vi "Analysis.Result Summaries, First and Last Pass Yield Paretos, Metrics Table.vi"(11 "ResultSum":T2[](array[typedef])) -> (0 "To Date":timestamp, 1 "From Date":timestamp, 2 "Test Count Table":string[][](table), 3 "Failure Pareto":string[][](table), 4 "LP Times Hist":T1(graph), 5 "Metrics Table":string[][](table), 6 "FP Times Hist":T1(graph), 7 "Durs":string[][](table))   [LabVIEW 2024]
uses:
  Analysis.Result Summary.ctl
panel:
  out "Tst Cnts":i32
  out "SNs":i32
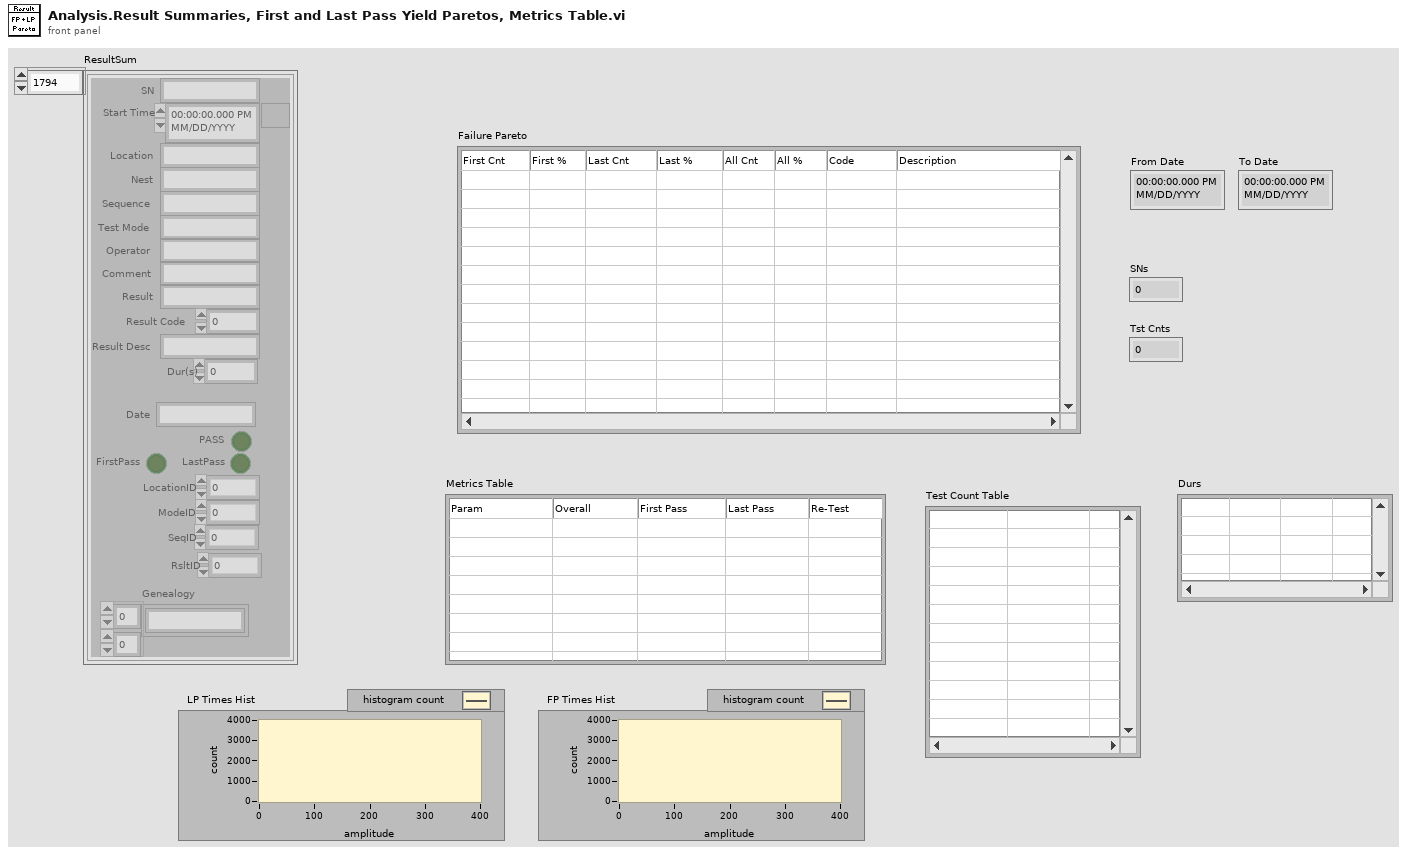
[diagram p1: front panel]
types:
  T1 = cluster{"X Values":dbl[], "Histogram: h(x)":i32[]}
  T2 = typedef "Analysis.Result Summary.ctl" = cluster{"SN":string, "Start Time":timestamp, "Location":string, "Nest":string, "Sequence":string, "Operator":string, "Test Mode":string, "Comment":string, "Result":string, "Result Code":i32, "Result Desc":string, "Date":string, "Dur(s)":dbl, "PASS":bool, "FirstPass":bool, "LastPass":bool, "LocationID":i32, "ModeID":i32, "SeqID":i32, "RsltID":i32, "Genealogy":string[][]}
  T3 = typedef "Analysis.Result Summary, Metrics.ctl" = cluster{"Pass Cnt":i32, "Fail Cnt":i32, "Yield%":dbl, "Test Cnt":i32, "SN Cnt":i32}
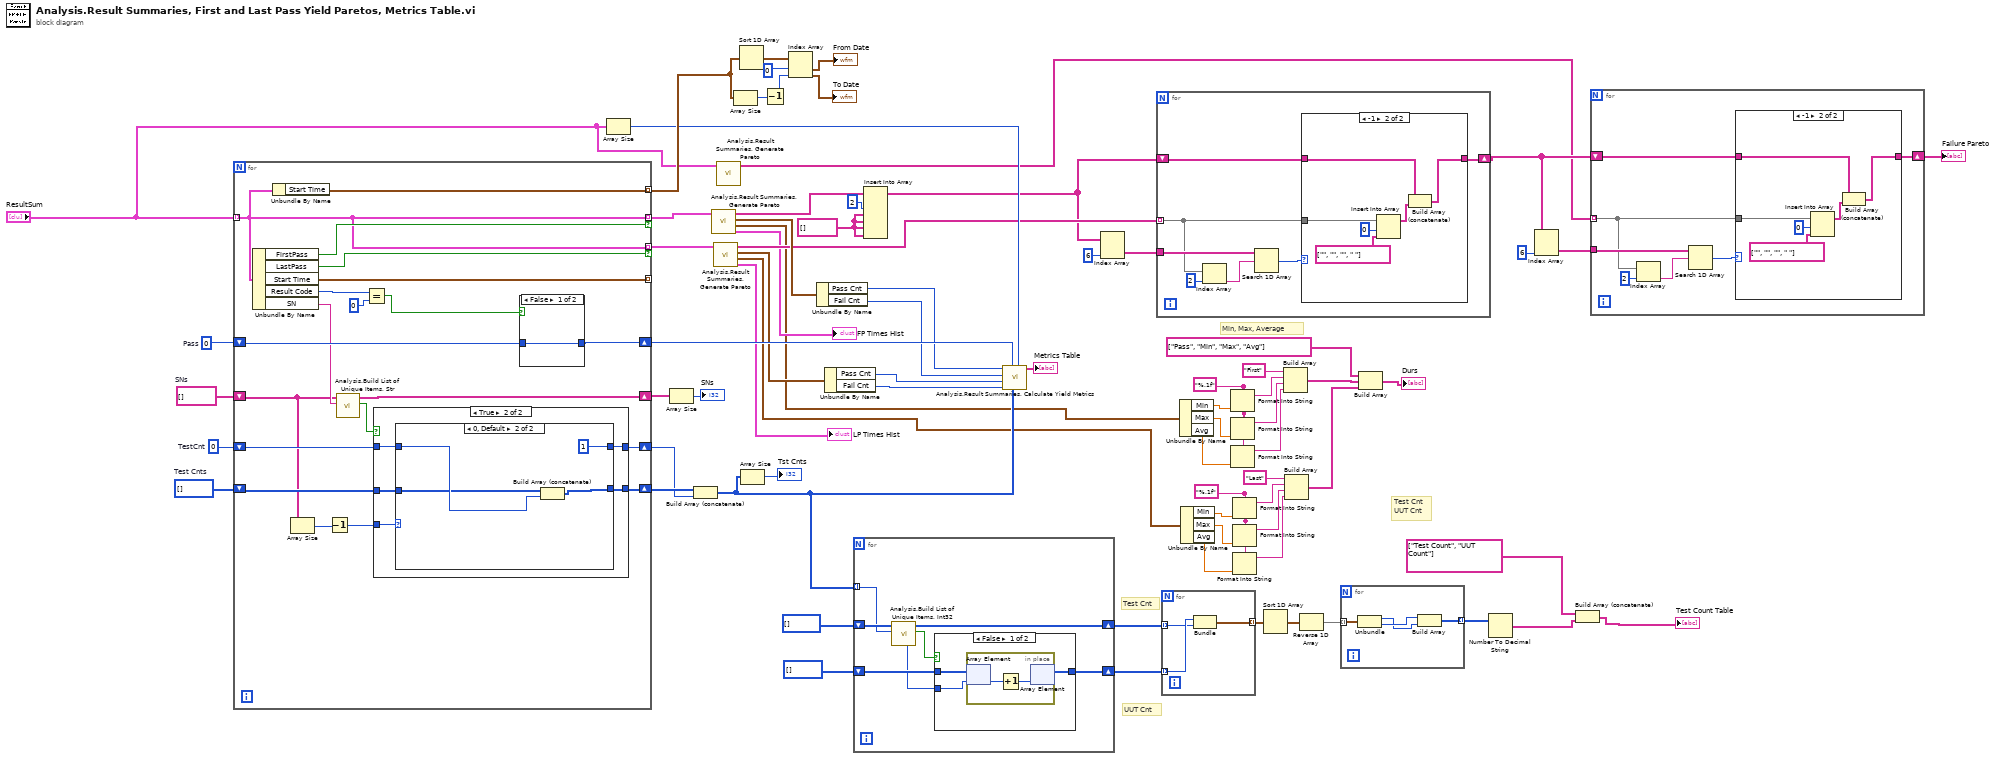
[diagram p0: block diagram]
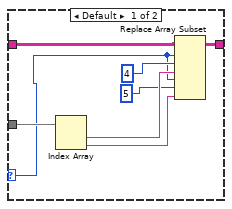
[diagram p2: hidden frame]
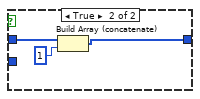
[diagram p3: hidden frame]
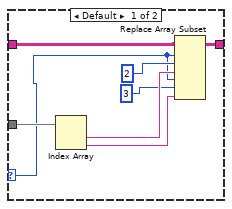
[diagram p4: hidden frame]
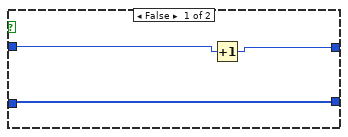
[diagram p5: hidden frame]
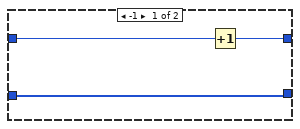
[diagram p6: hidden frame]
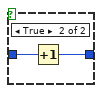
[diagram p7: hidden frame]
diagram:
  w17 = "%.1f"
  w24 = "%.1f"
  w6 = string[] []
  w65 = string[] []  # SNs
  w67 = i32[] []  # Test Cnts
  w66 = 0  # TestCnt
  w68 = 0  # Pass
  # "Min, Max, Average"
  # "Test Cnt\nUUT Cnt"
  # "Test Cnt"
  # "UUT Cnt"
  n1 = for {
    tunnel: "ResultSum" -> [w93] mode=indexing
    tunnel: [w93] -> w43 mode=indexing if=w96
    tunnel: [w93] -> w70 mode=indexing if=w95
    tunnel: [w94] -> _ mode=indexing
    tunnel: [w92] -> w69 mode=indexing
    shift-right: [w89] -> w63
    shift-left: w68 -> [w87]
    shift-right: [w81] -> w64
    shift-left: w67 -> [w83]
    shift-right: [w82] -> w54
    shift-left: w66 -> [w80]
    shift-right: [w85] -> w53
    shift-left: w65 -> [w79]
    n2 = Unbundle By Name(w93) -> ("FirstPass"=w96:bool, "LastPass"=w95:bool, "Start Time"=w94:timestamp, "Result Code"=w91:i32, "SN"=w86:string)
    n3 = Unbundle By Name(w93) -> ("Start Time"=w92:timestamp)
    n4 = Array Size(array=w79) -> (size(s)=w78:i32)
    n5 = Decrement(x=w78) -> (x-1=w77:i32)
    n6 = call "Analysis.Build List of Unique Items, Str.vi"("Item In"=w86, "List In"=w79) -> ("Added"=w84:bool, "List Out"=w85:string[])  [unwired: 7 in, 1 out]
    n7 = Equal?(x=w91, y=0) -> (x = y?=w88:bool)
    n8 = case shown="True" w84 {
      tunnel: w83 -> [w99 w101]
      tunnel: w80 -> [w98 w102]
      tunnel: [w97 w104] -> w82
      tunnel: [w99 w103] -> w81
      tunnel: w77 -> [_ w100]
      frame False {
        n9 = Increment(x=w98) -> (x+1=w97:i32)
      }
      frame True {
        n10 = case shown="0, Default" w100 {
          tunnel: [w105 1] -> w104
          tunnel: [w107 w110] -> w103
          tunnel: w102 -> [w106 w109]
          tunnel: w101 -> [w107 w108]
          frame -1 {
            n11 = Increment(x=w106) -> (x+1=w105:i32)
          }
          frame 0, Default {
            n12 = Build Array (concatenate)(w108, w109) -> (w110:i32[])
          }
        }
      }
    }
    n13 = case shown="False" w88 {
      tunnel: w87 -> [w112 w114]
      tunnel: [w112 w113] -> w89
      frame False {
      }
      frame True {
        n14 = Increment(x=w114) -> (x+1=w113:i32)
      }
    }
  }
  n15 = Array Size(array="ResultSum") -> (size(s)=w62:i32)
  n16 = Array Size(array=w53) -> (size(s)=→"SNs":i32)
  n17 = Build Array (concatenate)(w64, w54) -> (w44:i32[])
  n18 = call "Analysis.Result Summaries, Generate Pareto.vi"("ResultSum"=w43) -> ("Test Time Histogram"=→"FP Times Hist":T1, "Test Times (s)"=w28:cluster{"Min":dbl, "Max":dbl, "Avg":dbl}, "Metrics"=w61:T3, "FP Pareto"=w49:string[][])  [unwired: 7 in]
  n19 = call "Analysis.Result Summaries, Generate Pareto.vi"("ResultSum"=w70) -> ("Test Time Histogram"=→"LP Times Hist":T1, "Test Times (s)"=w8:cluster{"Min":dbl, "Max":dbl, "Avg":dbl}, "Metrics"=w58:T3, "FP Pareto"=w50:string[][])  [unwired: 7 in]
  n20 = call "Analysis.Result Summaries, Generate Pareto.vi"("ResultSum"="ResultSum") -> ("FP Pareto"=w1:string[][])  [unwired: 7 in, 3 out]
  n21 = Array Size(array=w69) -> (size(s)=w75:i32)
  n22 = Sort 1D Array(array=w69) -> (sorted array=w71:timestamp[])
  n23 = Array Size(array=w44) -> (size(s)=→"Tst Cnts":i32)
  n24 = Decrement(x=w75) -> (x-1=w74:i32)
  n25 = Index Array(array=w71, index #1=0 ("index"), index #2=w74) -> (element #1=→"From Date":timestamp, element #2=→"To Date":timestamp)
  n26 = Unbundle By Name(w61) -> ("Pass Cnt"=w60:i32, "Fail Cnt"=w59:i32)
  n27 = Unbundle By Name(w58) -> ("Pass Cnt"=w57:i32, "Fail Cnt"=w56:i32)
  n28 = for {
    tunnel: w44 -> [w119] mode=indexing
    shift-right: [w120] -> w40
    shift-left: i32[] [] ("Test Cnts") -> [w121]
    shift-right: [w116] -> w39
    shift-left: i32[] [] ("Test Cnts") -> [w117]
    n29 = call "Analysis.Build List of Unique Items, Int32.vi"("Item In"=w119, "List In"=w121) -> ("Added"=w118:bool, "List Out"=w120:i32[], "Index"=w115:i32)  [unwired: 7 in]
    n30 = case shown="False" w118 {
      tunnel: w117 -> [w124 w128]
      tunnel: [w123 w129] -> w116
      tunnel: w115 -> [w122 _]
      frame False {
        n31 = in-place {
          n32 = in-place-array #1(w124, w122) -> (w126:i32)
          n33 = Increment(x=w126) -> (x+1=w125:i32)
          n34 = in-place-array #1(w125) -> (w123:i32[])  [unwired: 1 out]
        }
      }
      frame True {
        n35 = Build Array (concatenate)(w128, 1) -> (w129:i32[])
      }
    }
  }
  n36 = Insert Into Array(array=w49, index (col)=2 ("index (row)"), new element #1=w6, new element #2=w6, new element #3=w6, new element #4=w6) -> (w48:string[][])  [unwired: 1 in]
  n37 = call "Analysis.Result Summaries, Calculate Yield Metrics.vi"("Total Cnt"=w62, "Retries"=w44, "Pass Cnt"=w63, "LP Fail"=w56, "LP Pass"=w57, "FP Fail"=w59, "FP Pass"=w60) -> ("Metrics Table"=→"Metrics Table":string[][])  [unwired: 4 in]
  n38 = Index Array(array=w48, index (col)=6 ("index (row)")) -> (element=w46:string[])  [unwired: 1 in]
  n39 = for {
    tunnel: w50 -> [w131] mode=indexing
    tunnel: w46 -> [w135]
    shift-right: [w130] -> w2
    shift-left: w48 -> [w133]
    n40 = Index Array(array=w131, index=2) -> (element=w134:string)
    n41 = Search 1D Array(1D array=w135, element=w134) -> (index of element=w132:i32)  [unwired: 1 in]
    n42 = case shown="-1" w132 {
      selector: w132 -> [w139 _]
      tunnel: w133 -> [w142 w150]
      tunnel: w131 -> [w144 w149]
      tunnel: [w143 w145] -> w130
      frame Default {
        n43 = Index Array(array=w144) -> (element #1=w140:string, element #2=w137:string)  [unwired: 2 in]
        n44 = Replace Array Subset(array=w142, new element #1=w140, index (row) #1=w139, index (col) #1=2 ("disabled index (col)"), new element #2=w137, index (row) #2=w139, index (col) #2=3 ("disabled index (col)")) -> (w143:string[][])
      }
      frame -1 {
        n45 = Insert Into Array(array=w149, index=0, new element=string[] ["", "", "", " "]) -> (w146:string[])
        n46 = Build Array (concatenate)(w150, w146) -> (w145:string[][])
      }
    }
  }
  n47 = for {
    tunnel: w40 -> [w152] mode=indexing
    tunnel: w39 -> [w153] mode=indexing
    tunnel: [w151] -> w38 mode=indexing
    n48 = Bundle("TestCnt"=w153, "TestCnt"=w152) -> (w151:cluster{"TestCnt":i32, "TestCnt":i32})  [unwired: 1 in]
  }
  n49 = Unbundle By Name(w28) -> ("Min"=w27:dbl, "Max"=w26:dbl, "Avg"=w25:dbl)
  n50 = Unbundle By Name(w8) -> ("Min"=w14:dbl, "Max"=w15:dbl, "Avg"=w16:dbl)
  n51 = Format Into String(format string=w24, w27) -> (resulting string=w23:string)  [unwired: 2 in, 1 out]
  n52 = Format Into String(format string=w24, w26) -> (resulting string=w22:string)  [unwired: 2 in, 1 out]
  n53 = Format Into String(format string=w24, w25) -> (resulting string=w21:string)  [unwired: 2 in, 1 out]
  n54 = Format Into String(format string=w17, w14) -> (resulting string=w18:string)  [unwired: 2 in, 1 out]
  n55 = Format Into String(format string=w17, w15) -> (resulting string=w19:string)  [unwired: 2 in, 1 out]
  n56 = Format Into String(format string=w17, w16) -> (resulting string=w20:string)  [unwired: 2 in, 1 out]
  n57 = Sort 1D Array(array=w38) -> (sorted array=w37:cluster{"TestCnt":i32, "TestCnt":i32}[])
  n58 = Build Array("First", w23, w22, w21) -> (w11:string[])
  n59 = Build Array("Last", w18, w19, w20) -> (w10:string[])
  n60 = Reverse 1D Array(array=w37) -> (reversed array=w36:cluster{"TestCnt":i32, "TestCnt":i32}[])
  n61 = for {
    tunnel: w36 -> [w157] mode=indexing
    tunnel: [w154] -> w35 mode=indexing
    n62 = Unbundle(w157) -> ("TestCnt"=w155:i32, "TestCnt"=w156:i32)
    n63 = Build Array(w156, w155) -> (w154:i32[])
  }
  n64 = Build Array(string[] ["Pass", "Min", "Max", "Avg"], w11, w10) -> (→"Durs":string[][])
  n65 = Number To Decimal String(number=w35) -> (decimal integer string=w32:string[][])  [unwired: 1 in]
  n66 = Index Array(array=w2, index (col)=6 ("index (row)")) -> (element=w5:string[])  [unwired: 1 in]
  n67 = Build Array (concatenate)(string[] ["Test Count", "UUT Count"], w32) -> (→"Test Count Table":string[][])
  n68 = for {
    tunnel: w1 -> [w159] mode=indexing
    tunnel: w5 -> [w163]
    shift-right: [w158] -> w3
    shift-left: w2 -> [w161]
    n69 = Index Array(array=w159, index=2) -> (element=w162:string)
    n70 = Search 1D Array(1D array=w163, element=w162) -> (index of element=w160:i32)  [unwired: 1 in]
    n71 = case shown="-1" w160 {
      selector: w160 -> [w167 _]
      tunnel: w161 -> [w170 w178]
      tunnel: w159 -> [w172 w177]
      tunnel: [w171 w173] -> w158
      frame Default {
        n72 = Index Array(array=w172) -> (element #1=w168:string, element #2=w165:string)  [unwired: 2 in]
        n73 = Replace Array Subset(array=w170, new element #1=w168, index (row) #1=w167, index (col) #1=4 ("disabled index (col)"), new element #2=w165, index (row) #2=w167, index (col) #2=5 ("disabled index (col)")) -> (w171:string[][])
      }
      frame -1 {
        n74 = Insert Into Array(array=w177, index=0, new element=string[] ["", "", "", " "]) -> (w174:string[])
        n75 = Build Array (concatenate)(w178, w174) -> (w173:string[][])
      }
    }
  }
  "Failure Pareto" <- w3
